vi "1D784_to_2D28_28_sub.vi"(1 "1D(784)":dbl[](array[numeric])) -> (0 "2D(28_28)":dbl[][](array[numeric]))   [LabVIEW 2021]
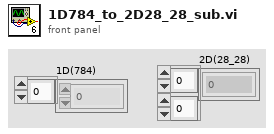
[diagram p1: front panel]
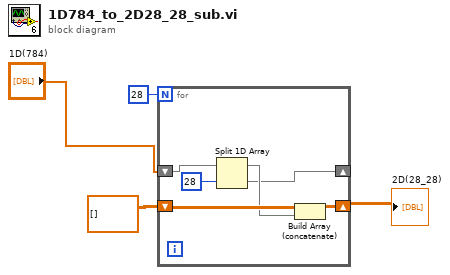
[diagram p0: block diagram]
diagram:
  n1 = for {
    N: 28 -> [_]
    shift-right: [w9] -> w1
    shift-left: dbl[][] [] -> [w8]
    shift-right: [w6] -> _
    shift-left: "1D(784)" -> [w5]
    n2 = Split 1D Array(array=w5, index=28) -> (first subarray=w7:dbl[], second subarray=w6:dbl[])
    n3 = Build Array (concatenate)(w8, w7) -> (w9:dbl[][])
  }
  "2D(28_28)" <- w1
